vi "Pre Launch Init.vi"(11 "Guardar Tipo CSV in":refnum<class "Guardar Tipo CSV.lvclass">) -> (0 "error out":errorcluster, 3 "Guardar Tipo CSV out":refnum<class "Guardar Tipo CSV.lvclass">)   [LabVIEW 2020, in "Guardar Tipo CSV.lvlib" / "Guardar Tipo CSV.lvclass"]
doc: "(<B>Filename</B>: Actor Framework.lvlib:Actor.lvclass:Pre Launch Init.vi)\n\nDefines behavior that occurs after the Launch Nested Actor method is invoked but before the actor's Actor Core method begins running.\n\nBy default, this method does nothing. A descendant class may override it to define behavior."
uses:
  Guardar Tipo CSV.lvclass
  <vilib>/ActorFramework/Actor/Actor.lvclass
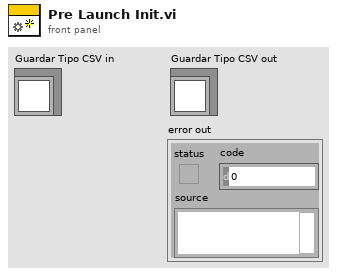
[diagram p1: front panel]
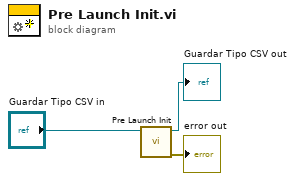
[diagram p0: block diagram]
diagram:
  n1 = call-parent "Pre Launch Init.vi"("Actor in"="Guardar Tipo CSV in") -> ("error out"=→"error out":errorcluster, "Actor out"=→"Guardar Tipo CSV out":refnum<class "Guardar Tipo CSV.lvclass">)  [unwired: 9 in]
